vi "TimeString.vi"() -> (0 "时间字符串":string)   [LabVIEW 2011]
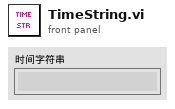
[diagram p1: front panel]
types:
  T1 = typedef "LVDateTimeRec.ctl" = cluster{"秒数的小数部分":dbl, "秒":i32, "分":i32, "时":i32, "日":i32, "月":i32, "年":i32, "天数（周）":i32, "天数（年）":i32, "DST":i32}
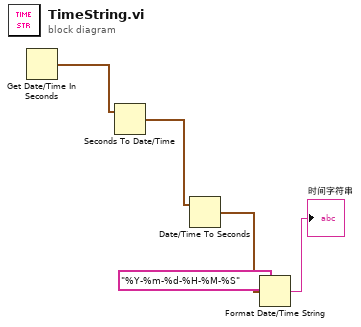
[diagram p0: block diagram]
diagram:
  n1 = Get Date/Time In Seconds() -> (seconds since 1Jan1904=w1:timestamp)
  n2 = Seconds To Date/Time(time stamp (now)=w1) -> (date time rec=w2:T1)  [unwired: 1 in]
  n3 = Date/Time To Seconds(2:w2) -> (0:w3:timestamp)  [unwired: 1 in]
  n4 = Format Date/Time String(time format string (%c)="%Y-%m-%d-%H-%M-%S" ("时间格式字符串(%c)"), seconds (now)=w3) -> (date/time string=→"时间字符串":string)  [unwired: 1 in]
